vi "Close.vi"(8 "error in (no error)":errorcluster, 11 "Carya Config in":refnum<class "Carya Config.lvclass">) -> (0 "error out":errorcluster)   [LabVIEW 2013, in "Carya Config.lvclass"]
doc: "Copyright 2018, Carya Automatisering, Wiebe Walstra."
uses:
  Carya Config.lvclass
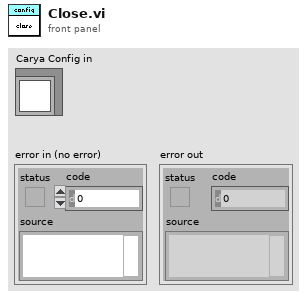
[diagram p1: front panel]
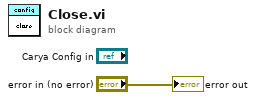
[diagram p0: block diagram]
diagram:
  "error out" <- "error in (no error)"
